vi "MFCLoop.vi"(8 "Error In":errorcluster, 10 "MFC Data":refnum<notifier>, 11 "Action Queues":T1) -> (0 "Error Out":errorcluster)   [LabVIEW 2012]
uses:
  ActionQueues.ctl
  UIActionQueueElement.ctl
  UIAction.ctl
  HardwareActionQueueElement.ctl
  HardwareAction.ctl
  HeaterActionQueueElement.ctl
  HeaterAction.ctl
  MFCActionQueueElement.ctl
  MFCAction.ctl
  LogActionQueueElement.ctl
  LogAction.ctl
  MFCConnectionData.ctl
  libs/Sierra-M100/Public/Controls/Gas.ctl
  libs/Sierra-M100/Public/Controls/Units.ctl
  <vilib>/Utility/error.llb/DialogType.ctl
  libs/Sierra-M100/Sierra-M100.lvlib
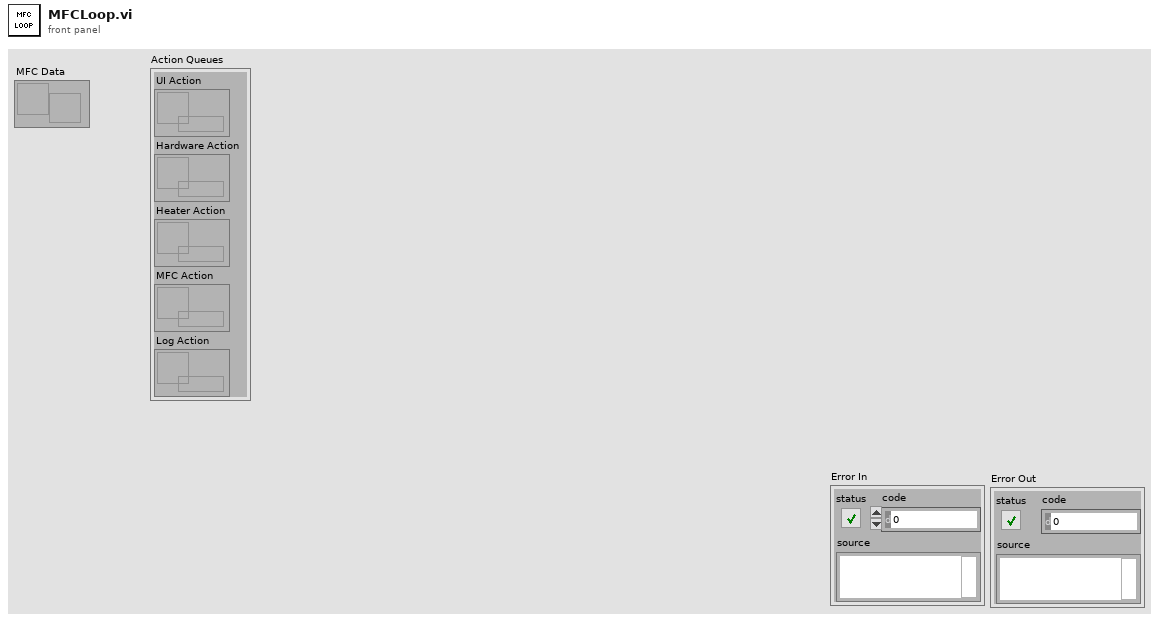
[diagram p1: front panel]
types:
  T1 = typedef "ActionQueues.ctl" = cluster{"UI Action":refnum<queue>, "Hardware Action":refnum<queue>, "Heater Action":refnum<queue>, "MFC Action":refnum<queue>, "Log Action":refnum<queue>}
  T2 = typedef "MFCActionQueueElement.ctl" = cluster{"Action":T3, "Data":variant}
  T3 = typedef "MFCAction.ctl" = enum16{"Initialize", "Start", "Read", "Write", "Stop", "Error", "Shutdown"}
  T4 = typedef "UIActionQueueElement.ctl" = cluster{"Action":T5, "Data":variant}
  T5 = typedef "UIAction.ctl" = enum16{"Initialize", "Connect", "MFC Connected", "Heater Connected", "Disconnect", "MFC Disconnected", "Heater Disconnected", "Configure MFC", "Configure Heater", "Open Log", "Close Log", "Shutdown"}
  T6 = typedef "MFCConnectionData.ctl" = cluster{"Name":string, "Firmware Version":string, "Serial Number":string, "Gas":T7, "Units":T8}
  T7 = typedef "Sierra-M100.lvlib/Gas.ctl" = enum16{"Air", "Argon", "CO2", "CO", "Helium", "Hydrogen", "Methane", "Nitrogen", "Nitrous Oxide", "Oxygen"}
  T8 = typedef "Sierra-M100.lvlib/Units.ctl" = enum16{"scc/s", "scc/m", "scc/H", "Ncc/s", "Ncc/m", "Ncc/H", "SCF/s", "SCF/m", "SCF/H", "NM3/s", "NM3/m", "NM3/H", "SM3/s", "SM3/m", "SM3/H", "sl/s", "sl/m", "sl/H", "NL/s", "NL/m", "Nl/H", "g/s", "g/m", "g/H", "kg/s", "kg/m", "kg/H", "lb/s", "lb/m", "lb/H"}
  T9 = typedef "DialogType.ctl" = u16
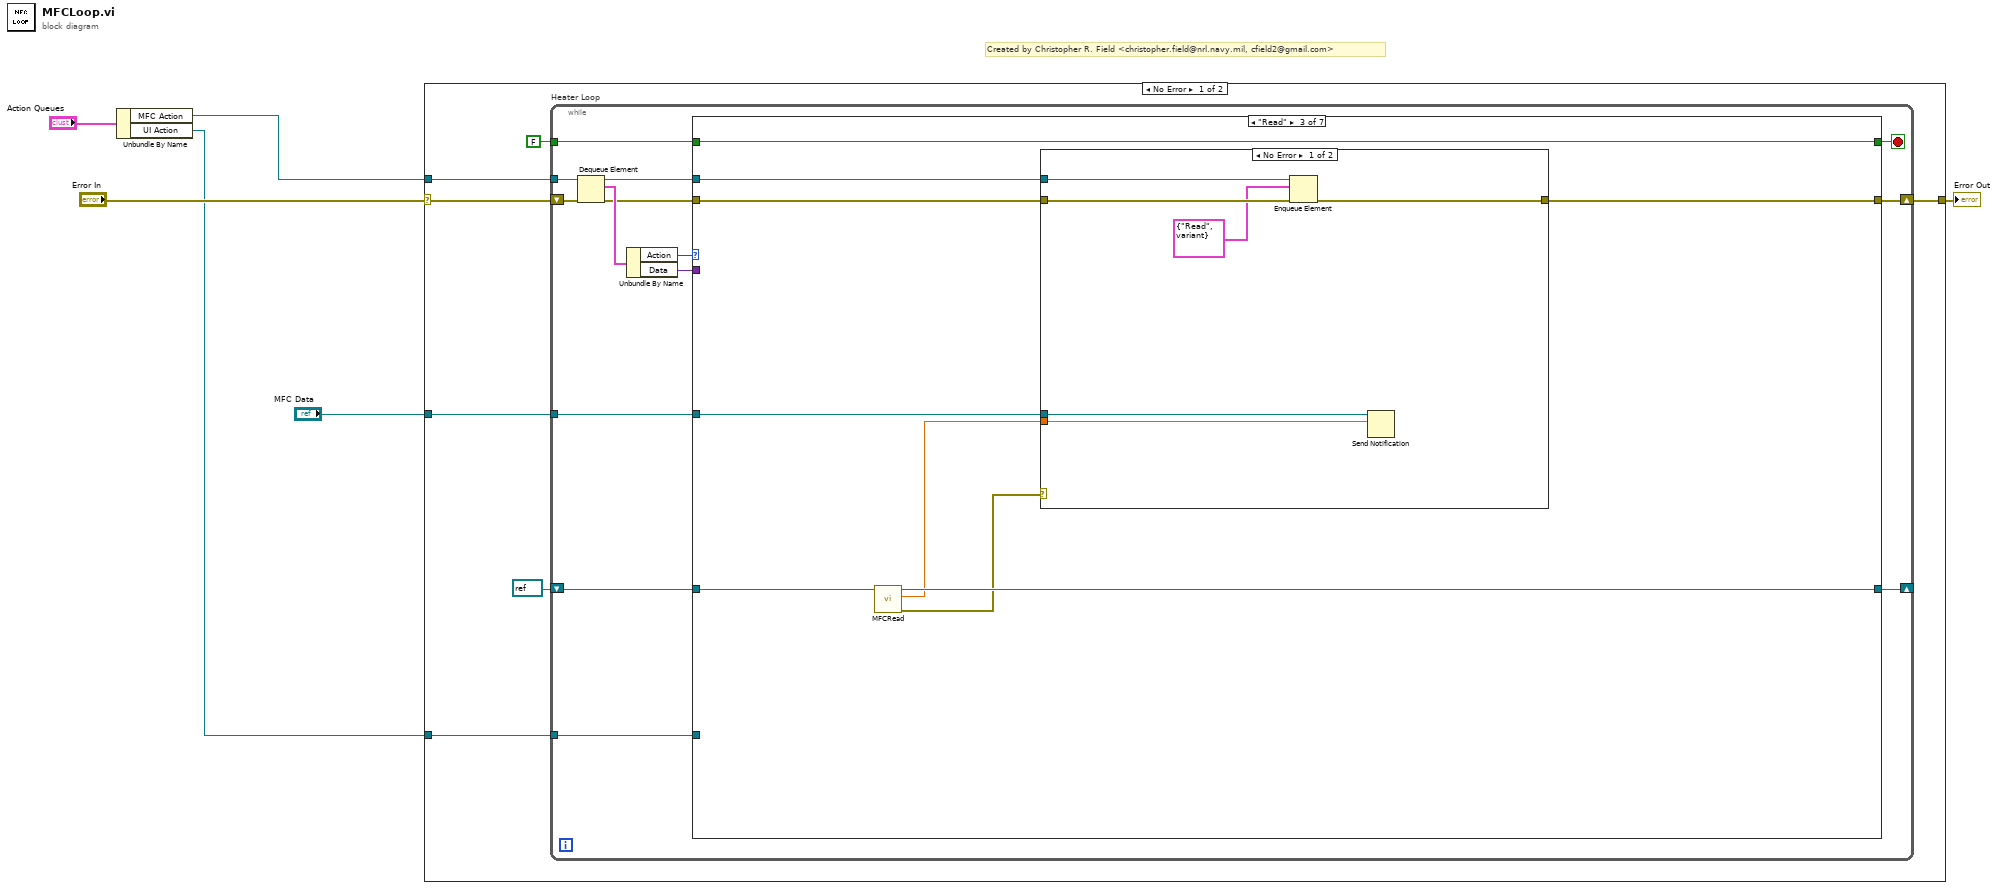
[diagram p0: block diagram]
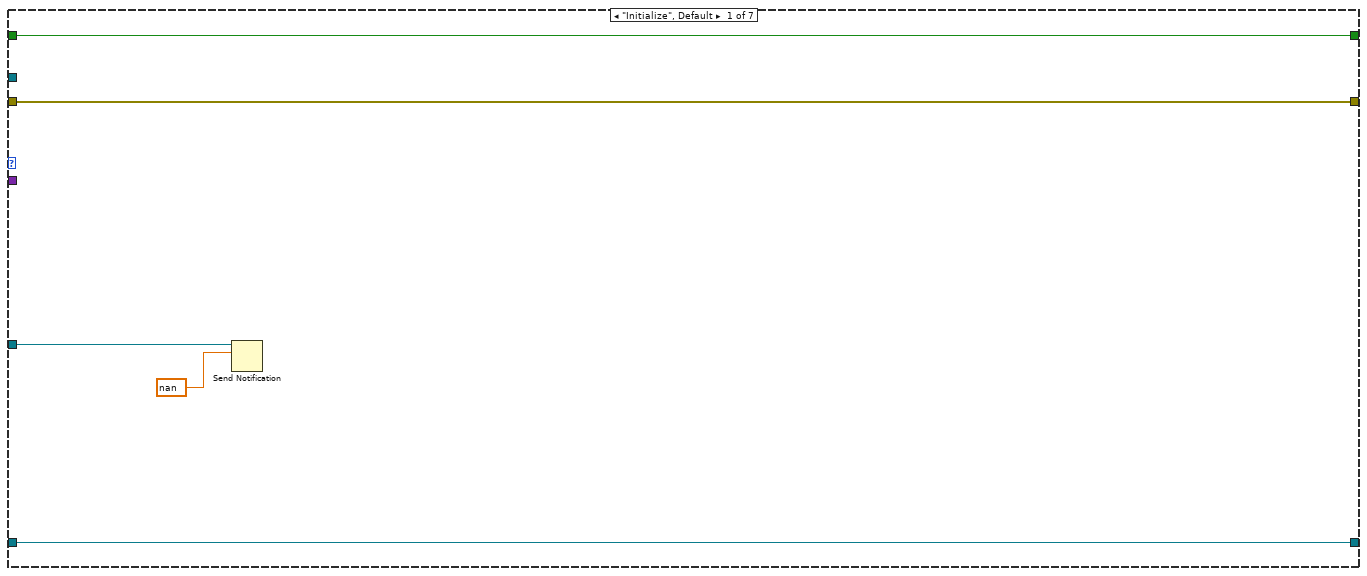
[diagram p2: hidden frame]
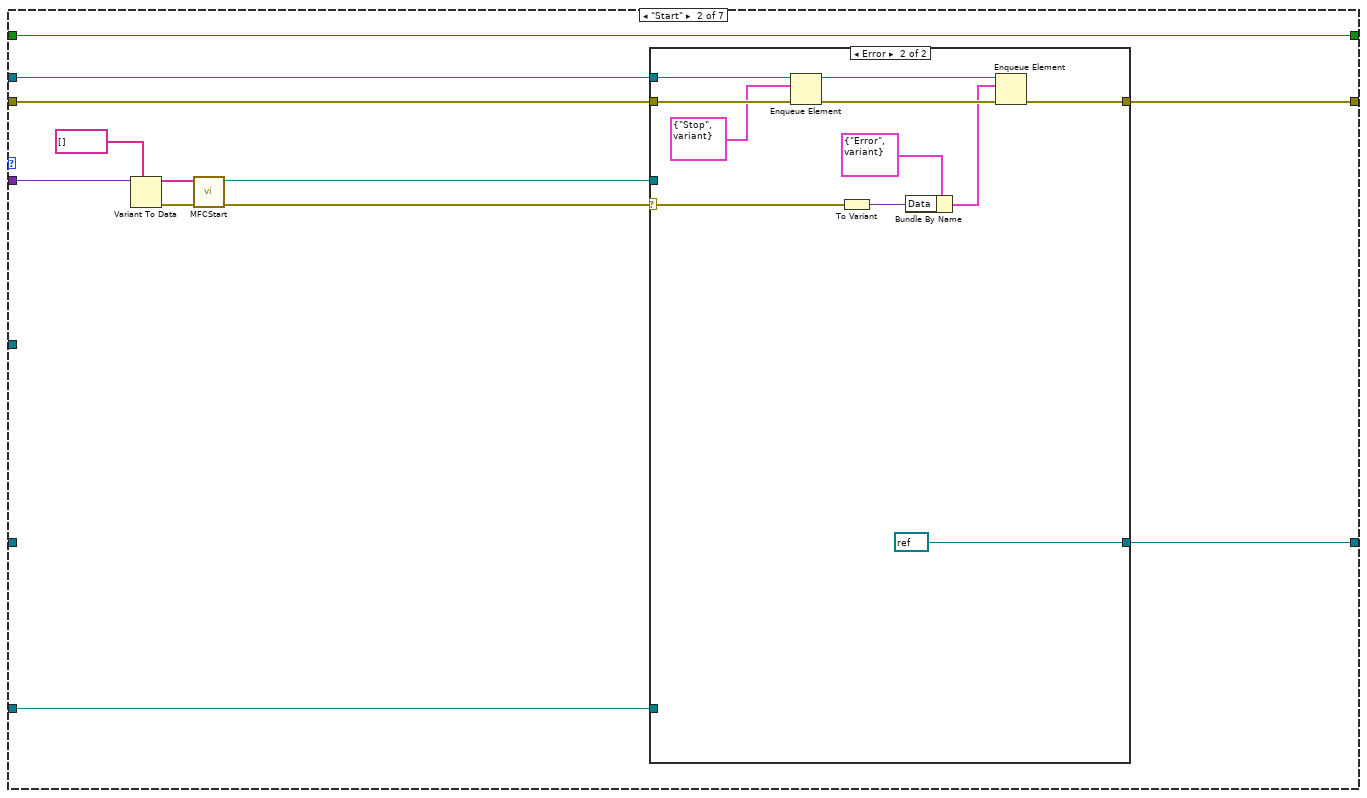
[diagram p3: hidden frame]
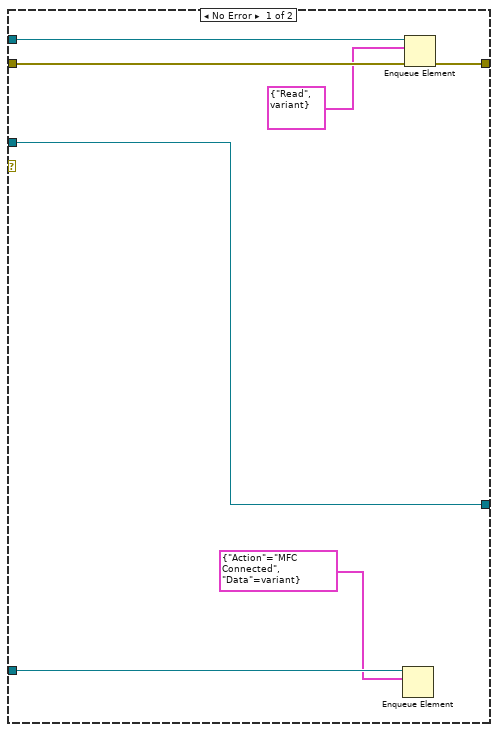
[diagram p4: hidden frame]
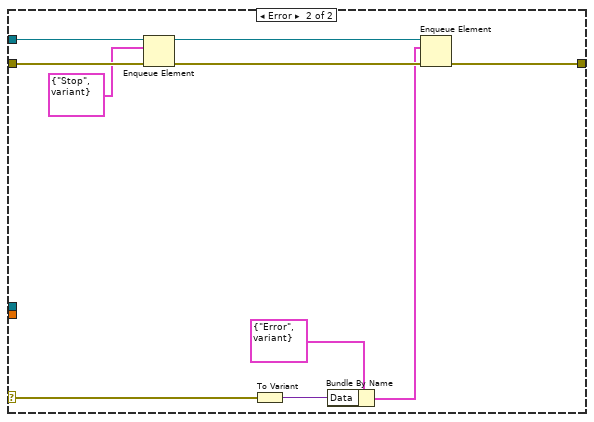
[diagram p5: hidden frame]
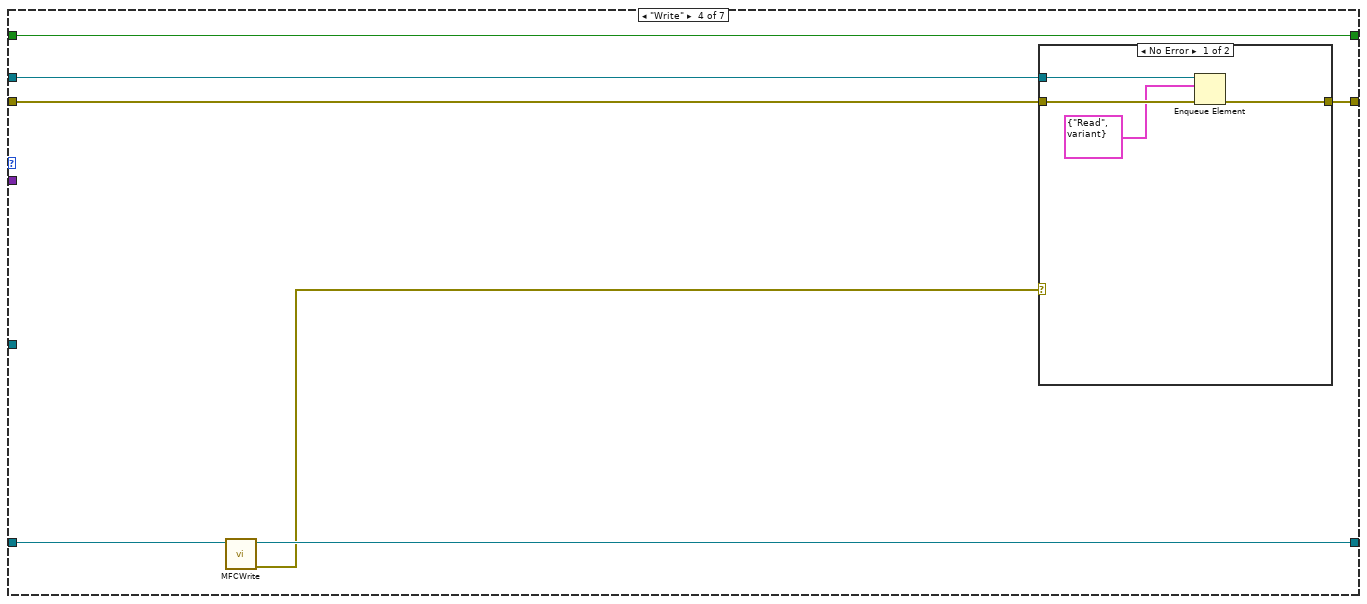
[diagram p6: hidden frame]
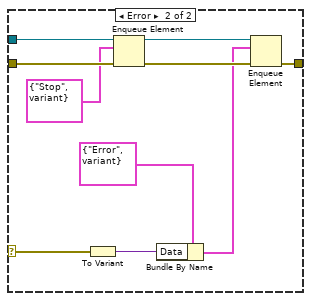
[diagram p7: hidden frame]
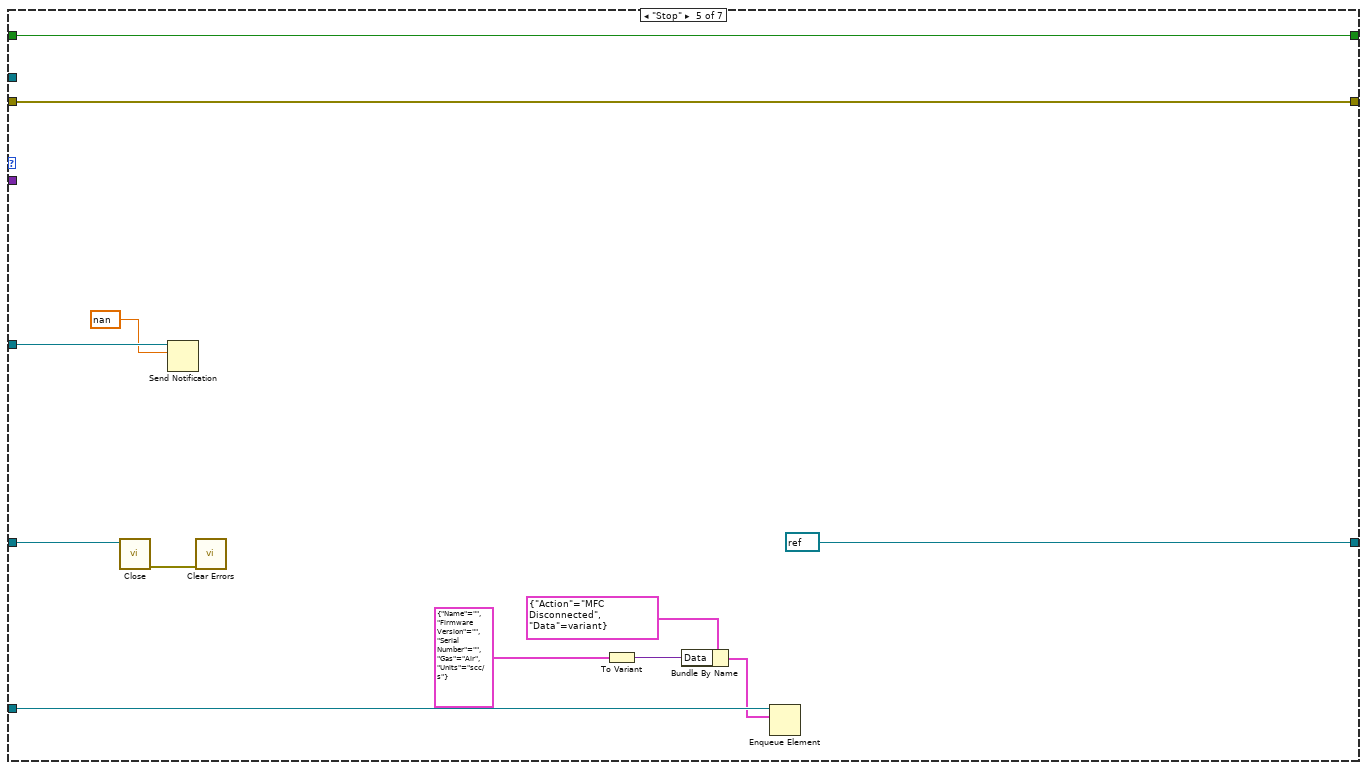
[diagram p8: hidden frame]
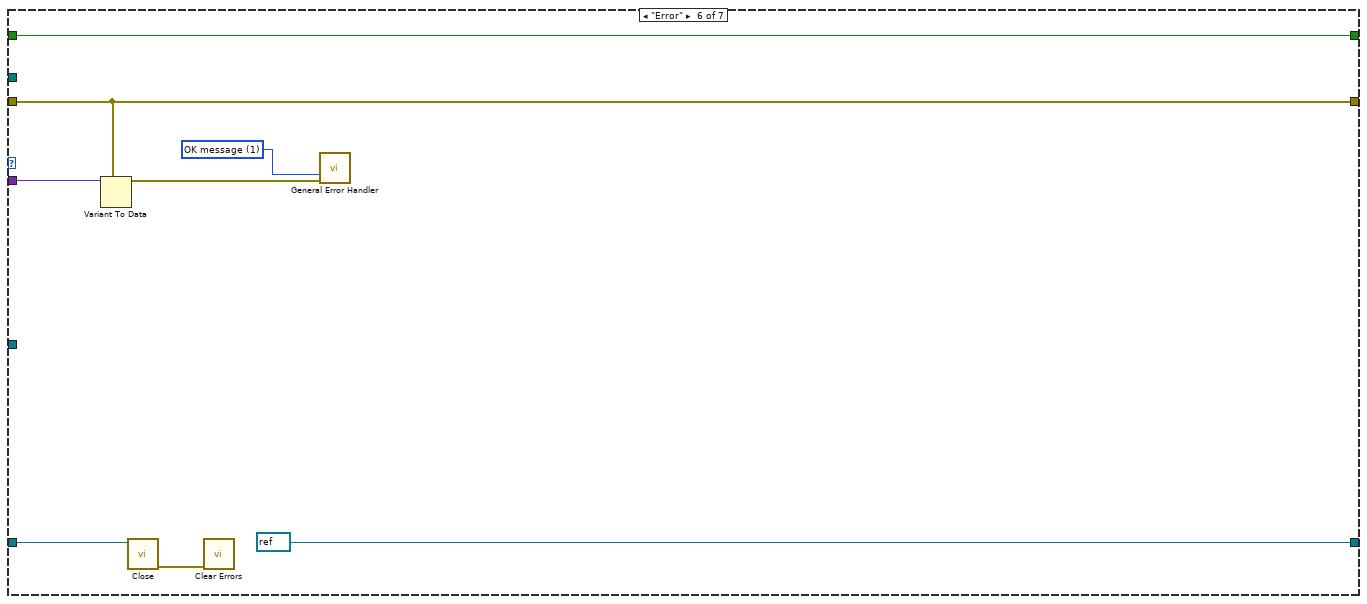
[diagram p9: hidden frame]
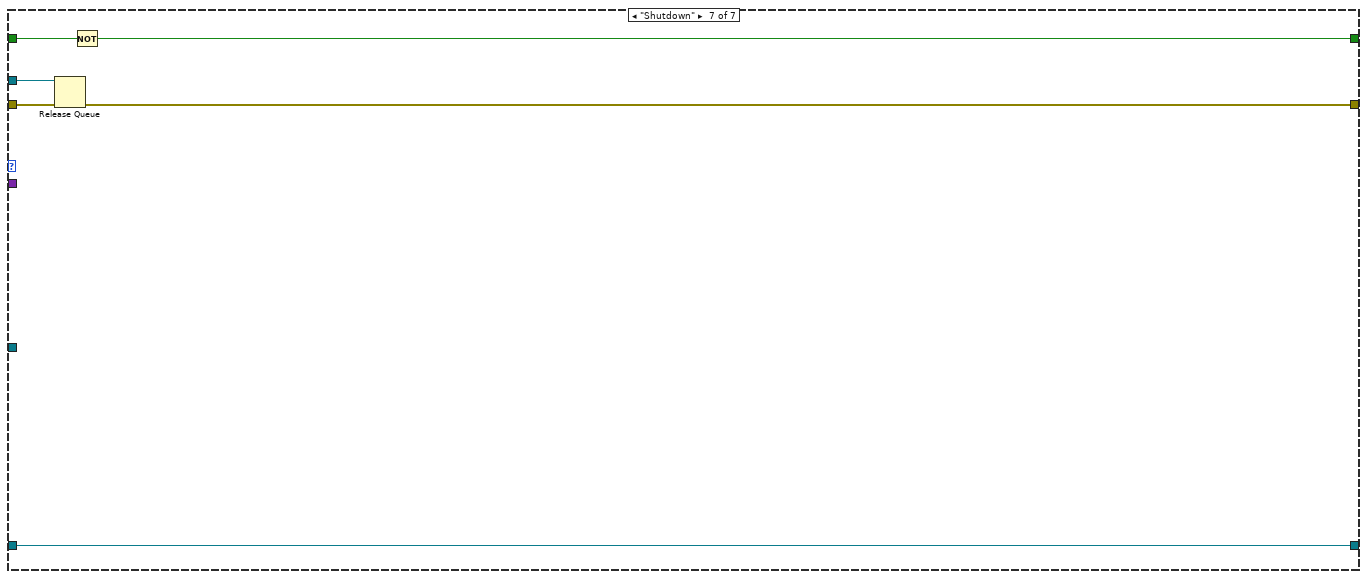
[diagram p10: hidden frame]
diagram:
  # "Created by Christopher R. Field <christopher.field@nrl.navy.mil, cfield2@gmail.com>"
  n1 = Unbundle By Name("Action Queues") -> ("MFC Action"=w3:refnum<queue>, "UI Action"=w2:refnum<queue>)
  n2 = case shown="No Error" "Error In" {
    selector: "Error In" -> [w12 w135]
    tunnel: [w11 w135] -> w5
    tunnel: w3 -> [w10 _]
    tunnel: "MFC Data" -> [w9 _]
    tunnel: w2 -> [w7 _]
    frame No Error {
      n3 = while "Heater Loop" {
        tunnel: FALSE -> [w27]
        shift-right: [w21] -> w11
        shift-left: w12 -> [w26]
        tunnel: w10 -> [w18]
        tunnel: w9 -> [w17]
        shift-right: [w16] -> _
        shift-left: refnum<visa-resource-name> refnum ("Smart Trak 2 Out") -> [w15]
        tunnel: w7 -> [w14]
        stop <- w19 stop-if-true
        n4 = Dequeue Element(queue=w18, error in (no error)=w26) -> (queue out=w20:refnum<queue>, element=w25:T2, error out=w22:errorcluster)  [unwired: 1 in, 1 out]
        n5 = Unbundle By Name(w25) -> ("Action"=w24:T3, "Data"=w23:variant)
        n6 = case shown="\"Read\"" w24 {
          tunnel: w27 -> [w31 w44 w71 w94 w120 w128 w134]
          tunnel: w23 -> [_ w38 _ _ _ w127 _]
          tunnel: w22 -> [w32 w41 w68 w92 w119 w126 w131]
          tunnel: [w32 w40 w67 w91 w119 w126 w130] -> w21
          tunnel: w20 -> [_ w39 w69 w93 _ _ w132]
          tunnel: [w31 w44 w71 w94 w120 w128 w133] -> w19
          tunnel: w17 -> [w30 _ w70 _ w116 _ _]
          tunnel: [w29 w42 w65 w89 refnum<visa-resource-name> refnum ("Smart Trak 2 Out") refnum<visa-resource-name> refnum ("Smart Trak 2 Out") w129] -> w16
          tunnel: w15 -> [w29 _ w66 w90 w118 w122 w129]
          tunnel: w14 -> [_ w43 _ _ w115 _ _]
          frame "Initialize", Default {
            n7 = Send Notification(notification=nan, notifier=w30) -> ()  [unwired: 1 in, 2 out]
          }
          frame "Start" {
            n8 = Variant To Data(type=string[] [] ("VISA Resources"), Variant=w38) -> (data=w36:string[], error out=w35:errorcluster)  [unwired: 1 in]
            n9 = call "MFCStart.vi"("Error In"=w35, "VISA Resource List"=w36) -> ("Error Out"=w34:errorcluster, "Sierra M100 Out"=w33:refnum<visa-resource-name>)  [unwired: 8 in]
            n10 = case shown="Error" w34 {
              selector: w34 -> [_ w52]
              tunnel: w43 -> [w51 _]
              tunnel: [w45 refnum<visa-resource-name> refnum ("Smart Trak 2 Out")] -> w42
              tunnel: w41 -> [w49 w60]
              tunnel: [w48 w57] -> w40
              tunnel: w39 -> [w50 w61]
              tunnel: w33 -> [w45 _]
              frame No Error {
                n11 = Enqueue Element(queue=w51, element=T4 {"Action"=enum."MFC Connected", "Data"=variant}) -> ()  [unwired: 2 in, 3 out]
                n12 = Enqueue Element(queue=w50, element=T2 {"Action"=enum."Read", "Data"=variant}, error in (no error)=w49) -> (error out=w48:errorcluster)  [unwired: 1 in, 2 out]
              }
              frame Error {
                n13 = Enqueue Element(queue=w61, element=T2 {"Action"=enum."Stop", "Data"=variant}, error in (no error)=w60) -> (queue out=w58:refnum<queue>, error out=w56:errorcluster)  [unwired: 1 in, 1 out]
                n14 = To Variant(anything=w52) -> (Variant=w54:variant)
                n15 = Bundle By Name(cluster=T2 {"Action"=enum."Error", "Data"=variant} ("element"), "Data"=w54) -> (w53:T2)
                n16 = Enqueue Element(queue=w58, element=w53, error in (no error)=w56) -> (error out=w57:errorcluster)  [unwired: 1 in, 2 out]
              }
            }
          }
          frame "Read" {
            n17 = call "MFCRead.vi"("Sierra M100 In"=w66) -> ("Error Out"=w64:errorcluster, "Flow Rate"=w63:dbl, "Sierra M100 Out"=w65:refnum<visa-resource-name>)  [unwired: 8 in]
            n18 = case shown="No Error" w64 {
              selector: w64 -> [_ w79]
              tunnel: w70 -> [w77 _]
              tunnel: w69 -> [w76 w87]
              tunnel: w68 -> [w75 w86]
              tunnel: [w74 w82] -> w67
              tunnel: w63 -> [w72 _]
              frame No Error {
                n19 = Enqueue Element(queue=w76, element=T2 {"Action"=enum."Read", "Data"=variant}, error in (no error)=w75) -> (error out=w74:errorcluster)  [unwired: 1 in, 2 out]
                n20 = Send Notification(notification=w72, notifier=w77) -> ()  [unwired: 1 in, 2 out]
              }
              frame Error {
                n21 = Enqueue Element(queue=w87, element=T2 {"Action"=enum."Stop", "Data"=variant}, error in (no error)=w86) -> (queue out=w84:refnum<queue>, error out=w83:errorcluster)  [unwired: 1 in, 1 out]
                n22 = To Variant(anything=w79) -> (Variant=w80:variant)
                n23 = Bundle By Name(cluster=T2 {"Action"=enum."Error", "Data"=variant} ("element"), "Data"=w80) -> (w78:T2)
                n24 = Enqueue Element(queue=w84, element=w78, error in (no error)=w83) -> (error out=w82:errorcluster)  [unwired: 1 in, 2 out]
              }
            }
          }
          frame "Write" {
            n25 = call "MFCWrite.vi"("Sierra M100 In"=w90) -> ("Error Out"=w88:errorcluster, "Sierra M100 Out"=w89:refnum<visa-resource-name>)  [unwired: 9 in]
            n26 = case shown="No Error" w88 {
              selector: w88 -> [_ w101]
              tunnel: w93 -> [w98 w108]
              tunnel: w92 -> [w97 w107]
              tunnel: [w95 w103] -> w91
              frame No Error {
                n27 = Enqueue Element(queue=w98, element=T2 {"Action"=enum."Read", "Data"=variant}, error in (no error)=w97) -> (error out=w95:errorcluster)  [unwired: 1 in, 2 out]
              }
              frame Error {
                n28 = To Variant(anything=w101) -> (Variant=w100:variant)
                n29 = Enqueue Element(queue=w108, element=T2 {"Action"=enum."Stop", "Data"=variant}, error in (no error)=w107) -> (queue out=w105:refnum<queue>, error out=w104:errorcluster)  [unwired: 1 in, 1 out]
                n30 = Bundle By Name(cluster=T2 {"Action"=enum."Error", "Data"=variant} ("element"), "Data"=w100) -> (w99:T2)
                n31 = Enqueue Element(queue=w105, element=w99, error in (no error)=w104) -> (error out=w103:errorcluster)  [unwired: 1 in, 2 out]
              }
            }
          }
          frame "Stop" {
            n32 = call "Close.vi"("Sierra M100 In"=w118) -> ("Error Out"=w110:errorcluster)  [unwired: 10 in]
            n33 = Send Notification(notification=nan, notifier=w116) -> ()  [unwired: 1 in, 2 out]
            n34 = call <vilib>:"Clear Errors.vi"("error in (no error)"=w110) -> ()  [unwired: 6 in, 1 out]
            n35 = To Variant(anything=T6 {"Name"="", "Firmware Version"="", "Serial Number"="", "Gas"=enum."Air", "Units"=enum."scc/s"} ("MFC Configuration Data")) -> (Variant=w113:variant)
            n36 = Bundle By Name(cluster=T4 {"Action"=enum."MFC Disconnected", "Data"=variant} ("element"), "Data"=w113) -> (w111:T4)
            n37 = Enqueue Element(queue=w115, element=w111) -> ()  [unwired: 2 in, 3 out]
          }
          frame "Error" {
            w124 = T9 1 items=["no dialog", "OK message", "continue or stop message", "OK message + warnings", "continue/stop + warnings"] ("type of dialog (OK msg:1)")
            n38 = Variant To Data(type=w126, Variant=w127) -> (data=w125:errorcluster)  [unwired: 1 in, 1 out]
            n39 = call "Close.vi"("Sierra M100 In"=w122) -> ("Error Out"=w123:errorcluster)  [unwired: 10 in]
            n40 = call <vilib>:"Clear Errors.vi"("error in (no error)"=w123) -> ()  [unwired: 6 in, 1 out]
            n41 = call <vilib>:"General Error Handler.vi"("type of dialog (OK msg:1)"=w124, "error in (no error)"=w125) -> ()  [unwired: 9 in, 5 out]
          }
          frame "Shutdown" {
            n42 = Release Queue(queue=w132, error in (no error)=w131) -> (error out=w130:errorcluster)  [unwired: 1 in, 2 out]
            n43 = Not(x=w134) -> (.not. x?=w133:bool)
          }
        }
      }
    }
    frame Error {
    }
  }
  "Error Out" <- w5
